vi "main.vi"() -> ()   [LabVIEW 2023]
uses:
  enum_read.ctl
  enum_readfile_loop.ctl
  enum_analyse.ctl
  enum_FGV.ctl
  Param in.ctl
panel:
  in  "Stop":bool
  in  "Tab Control":T1(tab)
  in  "Acq":bool
  in  "Tab Control 2":T2(tab)
  out "Order power spectrum":T3(graph)
  out "FFT Mag":cluster{"f0":dbl, "df":dbl, "magnitude":dbl[]}[](graph)
  out "Speed profile 2":cluster{"time [s]":dbl[], "speed [RPM]":dbl[]}(graph)
  out "przebieg czasowy":waveform(dbl)[](graph)
  out "Tryb maszyny":bool
  in  "Read file button":bool
  in  "Select file to read":path
  in  "Alarm order no. 2":dbl=155.5
  in  "Amplituda progu alarmowego (rząd) 2":dbl=2.0
  in  "Alarm order no. 1":dbl=155.5
  in  "Amplituda progu alarmowego (rząd)":dbl=2.0
  in  "axis1":i32=2
  in  "axis 2":i32=2
  out "Amplituda rzędu alarmowego 2":dbl
  out "Amplituda rzędu alarmowego":dbl
  in  "sampling frequency, Hz":dbl=1000.0
  in  "samples per channel":dbl
  # "Diagnostic application for cylindrical gear RCV 162/P"
  # "Analysis settings"
  # "Data input"
  # "alarm\namplitude"
  # "axis\nof interest"
  # "current\namplitude"
  # "User Manual for RCV 126/P Helical Gearbox Diagnostic Tool\n\nWelcome to the RCV 126/P Helical Gearbox Diagnostic Tool, a specialized app for monitoring the technical condition of your gearbox, capable of analyzing both real-time measurements and historical data from TDMS files. The app uses order analysis for precise diagnostics, displaying data in tabs on the main page including order power spectrum, FFT magnitude, speed profile, and the input signal.\n\n\nCustomization and operation\n\n         Data input - choose between real-time measurement or upload a TDMS file to begin analysis\n\n          Alarm configuration - user customization is our priority. The app allows you to set specific alarm orders and amplitudes based on your operational requirements. You can also choose the axis of interest (0 for X-axis, 1 for Y-axis, and 2 for Z-axis) to tailor the diagnostic focus to your specific needs.\n\n\nRecommended settings for RCV 162/P"
  # "Additional user settings"
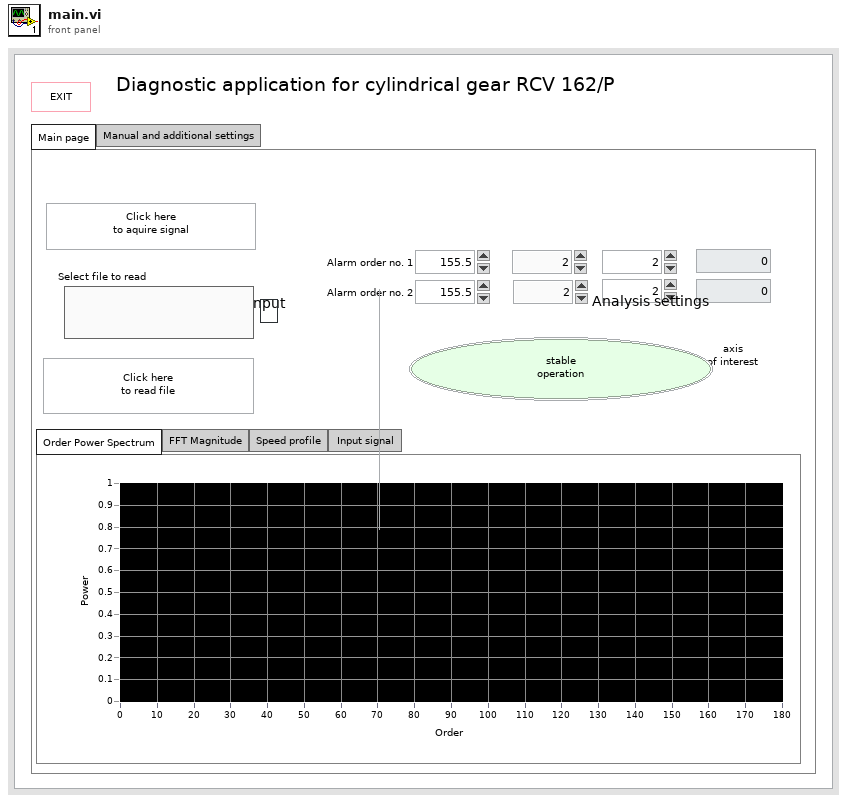
[diagram p1: front panel]
types:
  T1 = enum32{"Main page", "Manual and additional settings"}
  T2 = enum32{"Order Power Spectrum", "FFT Magnitude", "Speed profile", "Input signal "}
  T3 = cluster{"order 0":dbl, "delta order":dbl, "magnitude":dbl[]}[]
  T4 = typedef "enum_analyse.ctl" = enum16{"Idle", "Initialize", "Analyze", "End"}
  T5 = typedef "enum_readfile_loop.ctl" = enum16{"Idle", "Initialize", "Read_file", "End"}
  T6 = typedef "enum_read.ctl" = enum16{"Idle", "Init", "Read", "End"}
  T7 = typedef "enum_FGV.ctl" = enum16{"Get", "Set"}
  T8 = typedef "Param in.ctl" = cluster{"Acq":bool, "stop":bool, "Path":path, "rate":dbl, "s/ch":dbl, "Read":bool}
  T9 = typedef "Param out.ctl" = cluster{"Acq":bool, "stop":bool, "Path":path, "rate":dbl, "s/ch":dbl, "Read":bool}
  T10 = enum8{"Enabled", "Disabled", "Disabled and Grayed Out"}
  T11 = typedef "SoundVib_TachProcess.lvlib/speed profile.ctl" = cluster{"time [s]":dbl[], "speed [RPM]":dbl[]}
  T12 = cluster{"order 0":dbl, "delta order":dbl, "magnitude":dbl[]}
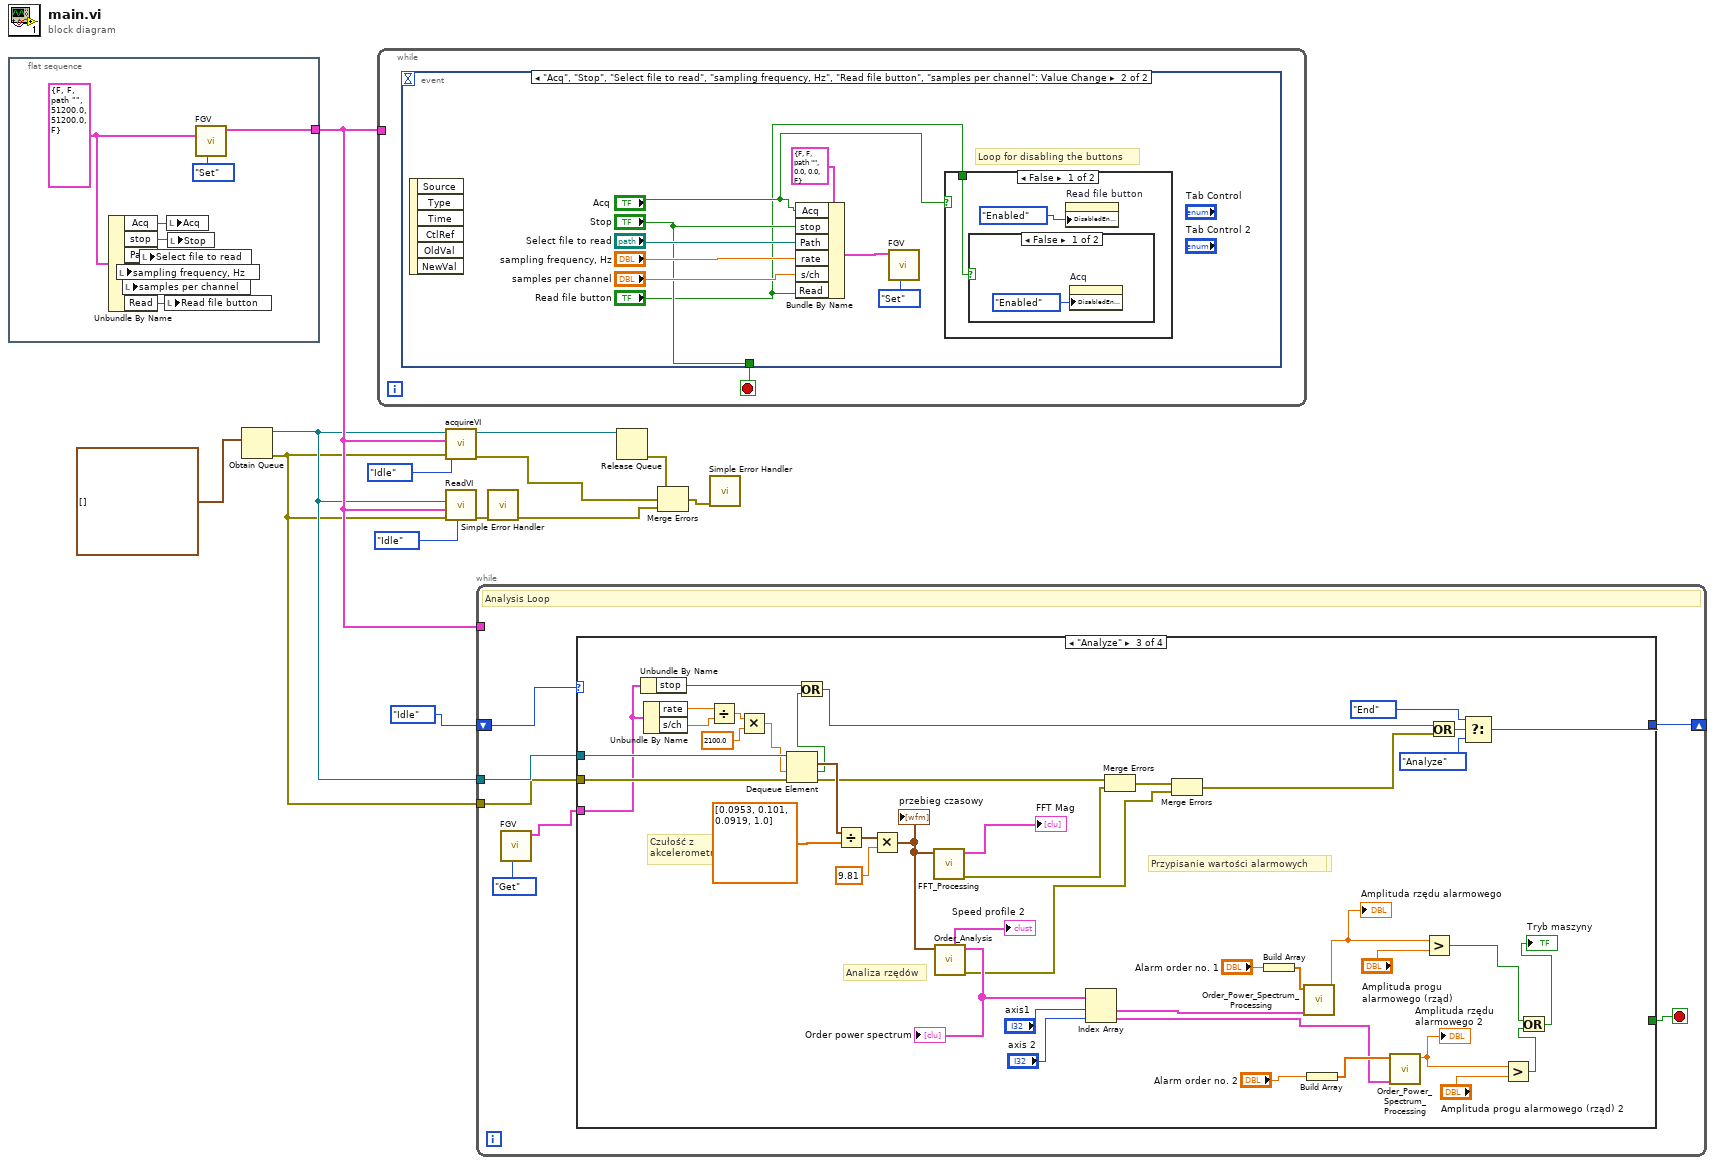
[diagram p0: block diagram]
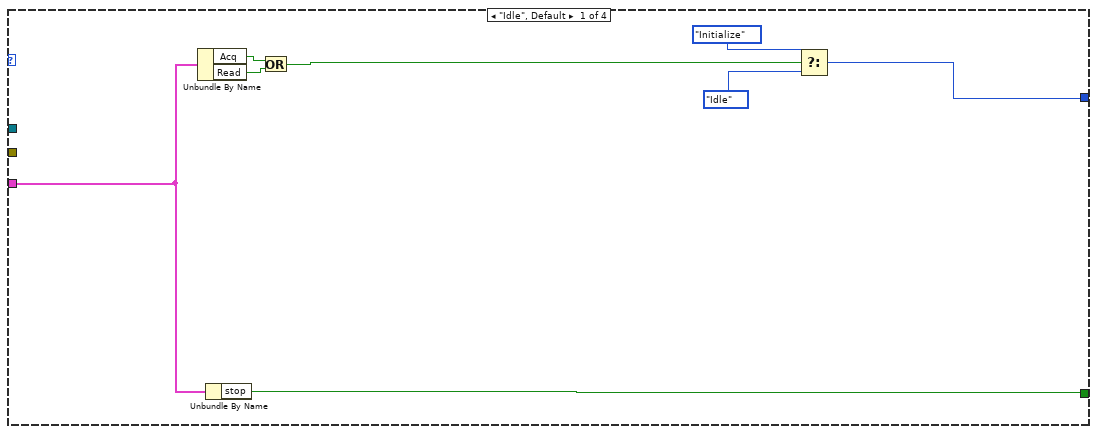
[diagram p2: hidden frame]
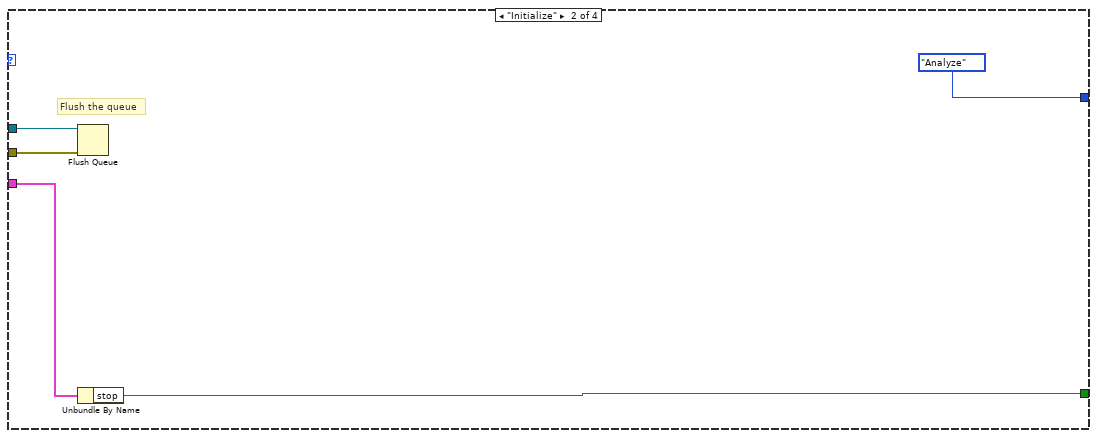
[diagram p3: hidden frame]
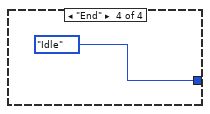
[diagram p4: hidden frame]
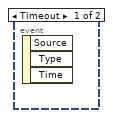
[diagram p5: hidden frame]
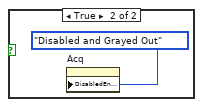
[diagram p6: hidden frame]
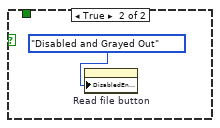
[diagram p7: hidden frame]
diagram:
  n1 = flat-sequence {
    tunnel: [w20] -> w7
    frame #0 {
      w22 = T8 {"Acq"=FALSE, "stop"=FALSE, "Path"=path "", "rate"=51200.0, "s/ch"=51200.0, "Read"=FALSE} ("Param in")
      n2 = Unbundle By Name(w22) -> ("Acq"=w19:bool, "stop"=w18:bool, "Path"=w17:path, "rate"=w16:dbl, "s/ch"=w15:dbl, "Read"=w14:bool)
      n3 = local write "sampling frequency, Hz"(w16) -> ()
      n4 = local write "samples per channel"(w15) -> ()
      n5 = local write "Select file to read"(w17) -> ()
      n6 = local write "Read file button"(w14) -> ()
      n7 = local write "Acq"(w19) -> ()
      n8 = local write "Stop"(w18) -> ()
      n9 = call "FGV.vi"("Action"=enum_FGV."Set", "Param in"=w22) -> ("Param out"=w20:T9)  [unwired: 9 in]
    }
  }
  n10 = Obtain Queue(element data type=waveform(dbl)[] [] ("data")) -> (queue out=w6:refnum<queue>, error out=w5:errorcluster)  [unwired: 4 in, 1 out]
  n11 = while {
    tunnel: w7 -> [_]
    stop <- w23 stop-if-true
    n12 = event shown="[1] \"Acq\", \"Stop\", \"Select file to read\", \"sampling frequency, Hz\", \"Read file button\", \"samples per channel\": Value Change" {
      selector: _ -> [_ _]
      dyn-events: _ -> [_ _]
      timeout: _ -> [_ _]
      tunnel: [_ "Stop"] -> w23
      event Timeout {
        n13 = event-data() -> ()  [unwired: 1 in, 3 out]
      }
      event "Acq", "Stop", "Select file to read", "sampling frequency, Hz", "Read file button", "samples per channel": Value Change {
        # "Loop for disabling the buttons"
        n14 = event-data() -> ()  [unwired: 1 in, 6 out]
        n15 = Bundle By Name(cluster=T8 {"Acq"=FALSE, "stop"=FALSE, "Path"=path "", "rate"=0.0, "s/ch"=0.0, "Read"=FALSE} ("Param in"), "Acq"="Acq", "stop"="Stop", "Path"="Select file to read", "rate"="sampling frequency, Hz", "s/ch"="samples per channel", "Read"="Read file button") -> (w31:T8)
        n16 = call "FGV.vi"("Action"=enum_FGV."Set", "Param in"=w31) -> ()  [unwired: 9 in, 1 out]
        n17 = case shown="False" "Acq" {
          tunnel: "Read file button" -> [w33 _]
          frame False {
            n18 = case shown="False" w33 {
              frame False {
                n19 = property on="Acq" class="Bool (strict)"("DisabledEnum"=T10."Enabled" ("Disabled")) -> ()  [unwired: 2 in, 2 out]
              }
              frame True {
                n20 = property on="Acq" class="Bool (strict)"("DisabledEnum"=T10."Disabled and Grayed Out" ("Disabled")) -> ()  [unwired: 2 in, 2 out]
              }
            }
            n21 = property on="Read file button" class="Bool (strict)"("DisabledEnum"=T10."Enabled" ("Disabled")) -> ()  [unwired: 2 in, 2 out]
          }
          frame True {
            n22 = property on="Read file button" class="Bool (strict)"("DisabledEnum"=T10."Disabled and Grayed Out" ("Disabled")) -> ()  [unwired: 2 in, 2 out]
          }
        }
      }
    }
  }
  n23 = call "acquireVI.vi"("error in (no error)"=w5, "Enum"=enum_read."Idle", "Param in"=w7, "Queue in"=w6) -> ("error out"=w3:errorcluster, "Queue out"=w11:refnum<queue>)  [unwired: 6 in]
  n24 = call "ReadVI.vi"("Enum"=enum_readfile_loop."Idle", "error in (no error)"=w5, "Param in"=w7, "queue in"=w6) -> ("error out"=w9:errorcluster)  [unwired: 7 in]
  n25 = while {
    tunnel: w7 -> [_]
    tunnel: w6 -> [w43]
    tunnel: w5 -> [w42]
    shift-right: [w38] -> _
    shift-left: enum_analyse."Idle" -> [w44]
    stop <- w39 stop-if-true
    # "Analysis Loop"
    n26 = call "FGV.vi"("Action"=enum_FGV."Get") -> ("Param out"=w40:T9)  [unwired: 10 in]
    n27 = case shown="\"Analyze\"" w44 {
      tunnel: w43 -> [_ w56 w94 _]
      tunnel: w42 -> [_ w55 w93 _]
      tunnel: w40 -> [w45 w53 w85 _]
      tunnel: [w46 w54 _ _] -> w39
      tunnel: [w47 enum_analyse."Analyze" w91 enum_analyse."Idle"] -> w38
      frame "Idle", Default {
        n28 = Unbundle By Name(w45) -> ("Acq"=w52:bool, "Read"=w51:bool)
        n29 = Unbundle By Name(w45) -> ("stop"=w46:bool)
        n30 = Or(x=w52, y=w51) -> (x .or. y?=w50:bool)
        n31 = Select(t=enum_analyse."Initialize", s=w50, f=enum_analyse."Idle") -> (s? t:f=w47:T4)
      }
      frame "Initialize" {
        # "Flush the queue"
        n32 = Flush Queue(queue=w56, error in (no error)=w55) -> ()  [unwired: 3 out]
        n33 = Unbundle By Name(w53) -> ("stop"=w54:bool)
      }
      frame "Analyze" {
        # "Decydowanie czy jest uszkodzenie"
        # "Przypisanie wartości alarmowych"
        # "Analiza rzędów"
        # "Czułość z akcelerometru"
        n34 = Unbundle By Name(w85) -> ("stop"=w81:bool)
        n35 = Unbundle By Name(w85) -> ("rate"=w87:dbl, "s/ch"=w86:dbl)
        n36 = Divide(x=w87, y=w86) -> (x/y=w84:dbl)
        n37 = Multiply(x=w84, y=2100.0) -> (x*y=w82:dbl)
        n38 = Dequeue Element(queue=w94, timeout in ms (-1)=w82, error in (no error)=w93) -> (element=w97:waveform(dbl)[], timed out?=w79:bool, error out=w95:errorcluster)  [unwired: 1 out]
        n39 = Or(x=w81, y=w79) -> (x .or. y?=w80:bool)
        n40 = Divide(x=w97, y=dbl[] [0.0953, 0.101, 0.0919, 1.0]) -> (x/y=w100:waveform(dbl)[])
        n41 = Multiply(x=w100, y=9.81) -> (x*y=w74:waveform(dbl)[])
        "przebieg czasowy" <- w74
        n42 = call "FFT_Processing.vi"("scaled signals [EU]"=w74) -> ("error out"=w72:errorcluster, "magnitudes [dB EU]"=→"FFT Mag":cluster{"f0":dbl, "df":dbl, "magnitude":dbl[]}[])  [unwired: 8 in, 1 out]
        n43 = call "Order_Analysis.vi"("array"=w74) -> ("error out"=w70:errorcluster, "order power spectra"=w77:T3, "speed profile"=→"Speed profile 2":T11)  [unwired: 8 in]
        "Order power spectrum" <- w77
        n44 = Index Array(array=w77, index #1="axis1", index #2="axis 2") -> (element #1=w69:T12, element #2=w59:T12)
        n45 = Merge Errors(w95, w72) -> (w96:errorcluster)
        n46 = Merge Errors(w96, w70) -> (w89:errorcluster)
        n47 = Build Array("Alarm order no. 1") -> (w60:dbl[])
        n48 = call "Order_Power_Spectrum_Processing.vi"("element"=w69, "magnitude"=w60) -> ("sum"=w75:dbl)  [unwired: 8 in, 1 out]
        "Amplituda rzędu alarmowego" <- w75
        n49 = Build Array("Alarm order no. 2") -> (w62:dbl[])
        n50 = call "Order_Power_Spectrum_Processing.vi"("element"=w59, "magnitude"=w62) -> ("sum"=w67:dbl)  [unwired: 8 in, 1 out]
        "Amplituda rzędu alarmowego 2" <- w67
        n51 = Greater?(x=w75, y="Amplituda progu alarmowego (rząd)") -> (0:w65:bool)
        n52 = Or(x=w80, y=w89) -> (x .or. y?=w90:bool)
        n53 = Select(t=enum_analyse."End", s=w90, f=enum_analyse."Analyze") -> (s? t:f=w91:T4)
        n54 = Greater?(x=w67, y="Amplituda progu alarmowego (rząd) 2") -> (0:w66:bool)
        n55 = Or(x=w65, y=w66) -> (x .or. y?=→"Tryb maszyny":bool)
      }
      frame "End" {
      }
    }
  }
  n56 = call <vilib>:"Simple Error Handler.vi"("error in (no error)"=w9) -> ("error out"=w4:errorcluster)  [unwired: 4 in, 4 out]
  n57 = Release Queue(queue=w11) -> (error out=w2:errorcluster)  [unwired: 2 in, 2 out]
  n58 = Merge Errors(w2, w3, w4) -> (w1:errorcluster)
  n59 = call <vilib>:"Simple Error Handler.vi"("error in (no error)"=w1) -> ()  [unwired: 4 in, 5 out]
